vi "TIO Device Init.vi"(9 "ID":string="Twinleaf", 11 "URL":refnum<visa-resource-name>="tcp://localhost") -> (0 "error out":errorcluster={"status"=TRUE, "code"=-1073807252, "source"="VISA Read in SLIP Decode Serial Read.vi->NN VISA Read.vi->NN RPC.vi"}, 1 "Connected":bool, 2 "ID Verified":bool, 3 "TIO":T1={"TS Connection"={"Type"=enum."Serial", "URL"="serial:///dev/cu.usbserial-00000", "TO"=500, "Addr"=0, "Port"=0, "TCP"=refnum, "UDP"=refnum, "Route"=""}, "REQ"=refnum, "REP"=refnum}, 4 "ID Verified":string)   [LabVIEW 2017]
uses:
  <instrlib>/tio-labview/TIO Library/TIO Serial Port Name Search.vi
  <instrlib>/tio-labview/TIO Library/TIO Stream Write.vi
  <instrlib>/tio-labview/TIO Library/TIO RPC Form Request.vi
  <instrlib>/tio-labview/TIO Library/TIO SLIP Serial Write.vi
  <instrlib>/tio-labview/TIO Library/TIO Form Packet.vi
  <instrlib>/tio-labview/TIO Library/TIO SLIP Encode.vi
  <instrlib>/tio-labview/TIO Library/TIO Serial Checksum CRC32.vi
  <vilib>/Instr/_visa.llb/VISA Configure Serial Port (Instr).vi
  <instrlib>/tio-labview/TIO Library/TIO Serial Port Discovery.vi
  <vilib>/Utility/tcp.llb/UDP Multicast Open.vi
  <vilib>/Utility/tcp.llb/UDP Multicast Read-Write Open.vi
panel:
  in  "RX Only":bool
  # "TIO Init"
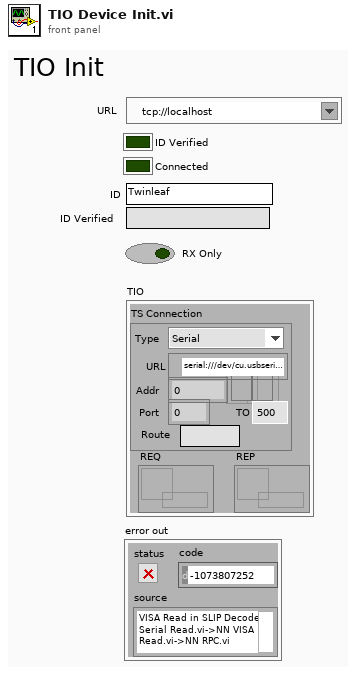
[diagram p1: front panel]
types:
  T1 = cluster{"TS Connection":cluster{"Type":enum16{"Serial", "TCP", "UDP", "mUDP"}, "URL":refnum<visa-resource-name>, "TO":u32, "Addr":u32, "Port":i32, "TCP":refnum<k5>, "UDP":refnum<k16>, "Route":string}, "REQ":refnum<queue>, "REP":refnum<queue>}
  T2 = cluster{"Type":enum16{"Serial", "TCP", "UDP", "mUDP"}, "URL":refnum<visa-resource-name>, "TO":u32, "Addr":u32, "Port":i32, "TCP":refnum<k5>, "UDP":refnum<k16>, "Route":string}
  T3 = cluster{"TC Connection":cluster{"Type":enum16{"Serial", "TCP", "UDP", "mUDP"}, "URL":refnum<visa-resource-name>, "TO":u32, "Addr":u32, "Port":i32, "TCP":refnum<k5>, "UDP":refnum<k16>, "Route":string}, "queue out":refnum<queue>, "queue out":refnum<queue>}
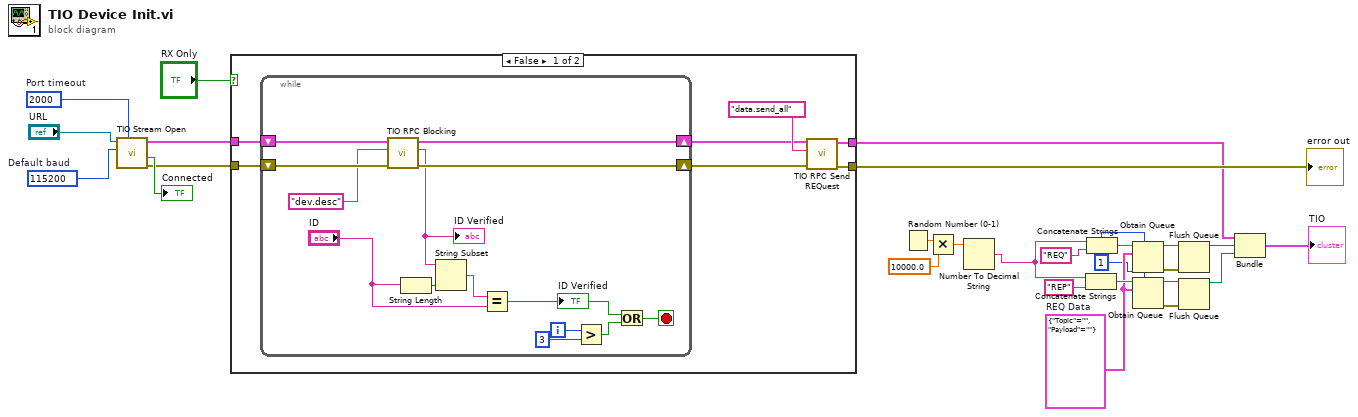
[diagram p0: block diagram]
diagram:
  w12 = u32 115200  # Default baud
  w11 = u32 2000  # Port timeout
  w18 = 1 ("max queue size (-1, unlimited)")
  w19 = cluster{"Topic":string, "Payload":string} {"Topic"="", "Payload"=""}  # REQ Data
  n1 = call <instrlib>:"TIO Stream Open.vi"("Port timeout"=w11, "Default baud"=w12, "URL"="URL") -> ("error out"=w7:errorcluster, "Connected"=→"Connected":bool, "TC Connection"=w8:T2)  [unwired: 6 in]
  n2 = case shown="False" "RX Only" {
    tunnel: [w33 w48] -> w26
    tunnel: [w32 w49] -> w13
    tunnel: w8 -> [w28 w49]
    tunnel: w7 -> [w27 w48]
    frame False {
      n3 = while {
        shift-right: [w46] -> w29
        shift-left: w28 -> [w45]
        shift-right: [w47] -> w30
        shift-left: w27 -> [w44]
        i -> [w38]
        stop <- w34 stop-if-true
        n4 = call <instrlib>:"TIO RPC Blocking.vi"("error in (no error)"=w44, "Named Method"="dev.desc" ("Topic"), "TC Connection"=w45) -> ("error out"=w47:errorcluster, "Respose"=w41:string, "TC Connection"=w46:T2)  [unwired: 5 in, 1 out]
        "ID Verified" <- w41
        n5 = String Length(string="ID") -> (length=w42:i32)
        n6 = String Subset(string=w41, length (rest)=w42) -> (substring=w40:string)  [unwired: 1 in]
        n7 = Equal?(x=w40, y="ID") -> (x = y?=w36:bool)
        "ID Verified" <- w36
        n8 = Greater?(x=w38, y=3) -> (0:w35:bool)
        n9 = Or(x=w36, y=w35) -> (x .or. y?=w34:bool)
      }
      n10 = call <instrlib>:"TIO RPC Send REQuest.vi"("error in (no error)"=w30, "Topic"="data.send_all", "TC Connection"=w29) -> ("error out"=w33:errorcluster, "TC Connection"=w32:T2)  [unwired: 6 in, 1 out]
    }
    frame True {
    }
  }
  "error out" <- w26
  n11 = Random Number (0-1)() -> (number: 0 to 1=w6:dbl)
  n12 = Multiply(x=w6, y=10000.0) -> (x*y=w4:dbl)
  n13 = Number To Decimal String(number=w4) -> (decimal integer string=w3:string)  [unwired: 1 in]
  n14 = Concatenate Strings(w3, "REP" ("name (unnamed)")) -> (w22:string)
  n15 = Concatenate Strings(w3, "REQ" ("name (unnamed)")) -> (w23:string)
  n16 = Obtain Queue(max queue size (-1, unlimited)=w18, name (unnamed)=w23, element data type=w19) -> (queue out=w21:refnum<queue>, error out=w20:errorcluster)  [unwired: 2 in, 1 out]
  n17 = Obtain Queue(max queue size (-1, unlimited)=w18, name (unnamed)=w22, element data type=w19) -> (queue out=w25:refnum<queue>, error out=w24:errorcluster)  [unwired: 2 in, 1 out]
  n18 = Flush Queue(queue=w21, error in (no error)=w20) -> (queue out=w15:refnum<queue>)  [unwired: 2 out]
  n19 = Flush Queue(queue=w25, error in (no error)=w24) -> (queue out=w14:refnum<queue>)  [unwired: 2 out]
  n20 = Bundle("TC Connection"=w13, "queue out"=w15, "queue out"=w14) -> (→"TIO":T3)  [unwired: 1 in]
